vi "Exemple_Extraction_FeatureHasher.vi"() -> ()   [LabVIEW 2020]
uses:
  Objet/6 - Datasets Transformation/6.2 - Feature extraction/FeatureHasher/FeatureHasher.lvclass
panel:
  in  "y":string[][](array[string])
  in  "X":string[][](array[string])
  in  "FeatureHasher":T1={"n_features"=1048576, "input_type"="dict", "dtype"="float", "alternate_sign"=TRUE}
  out "Data":T2
  out "error out":errorcluster caption="sortie d'erreur"
  in  "error in":errorcluster caption="entrée d'erreur"
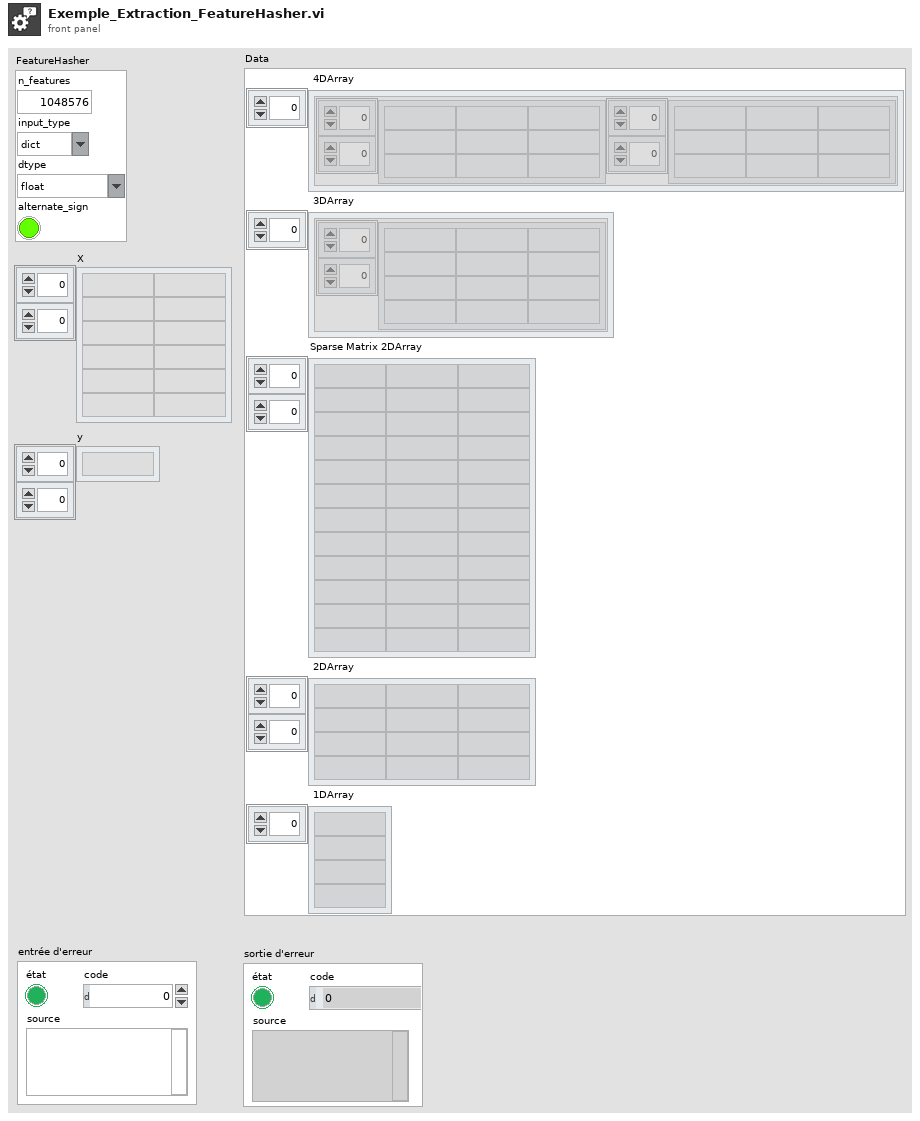
[diagram p1: front panel]
types:
  T1 = cluster{"n_features":i32, "input_type":string, "dtype":string, "alternate_sign":bool}
  T2 = cluster{" 4DArray":cluster{"1":string[][], "2":string[][]}[], " 3DArray":cluster{"Tableau":string[][]}[], "Sparse Matrix 2DArray":string[][], " 2DArray":string[][], " 1DArray":string[]}
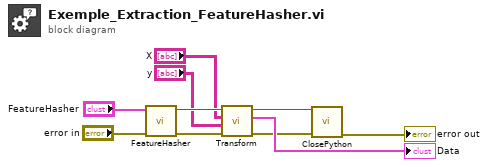
[diagram p0: block diagram]
diagram:
  n1 = call "FeatureHasher.vi"("error in"="error in", "FeatureHasher"="FeatureHasher") -> ("error out"=w6:errorcluster, "FeatureHasher.lvclass"=w7:refnum<class "FeatureHasher.lvclass">)  [unwired: 8 in]
  n2 = call-dynamic "Transform.vi"("error in (no error)"=w6, "y"="y", "X"="X", "FeatureHasher.lvclass"=w7) -> ("error out"=w3:errorcluster, "Data"=→"Data":T2, "FeatureHasher.lvclass"=w5:refnum<class "FeatureHasher.lvclass">)  [unwired: 5 in]
  n3 = call-dynamic "ClosePython.vi"("error in (no error)"=w3, "Scikit-learn en entrée"=w5) -> ("error out"=→"error out":errorcluster)  [unwired: 8 in, 1 out]
